vi "ResultsViewer.vi"(8 "Error in":errorcluster, 11 "TDMS path":path=path "") -> (0 "Error out":errorcluster)   [LabVIEW 2019]
panel:
  out "Loaded TDMS Filename":string
  out "O2 Saturation":dbl[](graph)
  out "Heart beat":dbl[](graph)
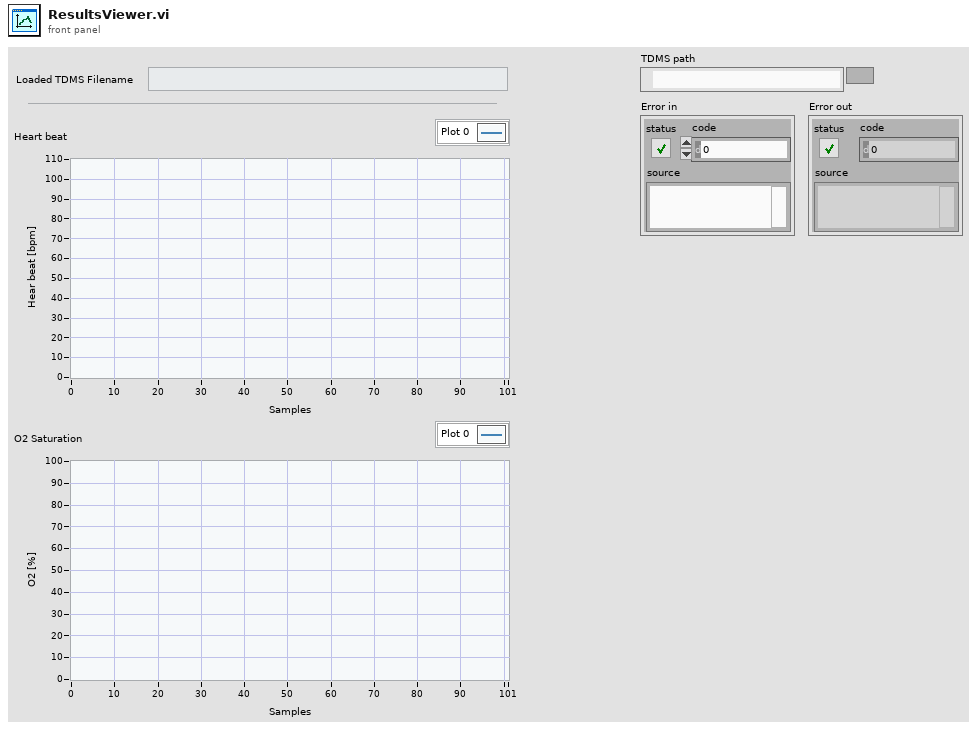
[diagram p1: front panel]
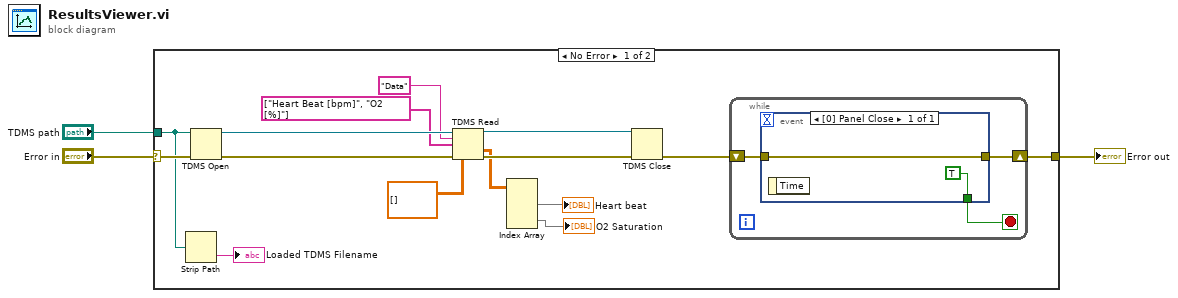
[diagram p0: block diagram]
diagram:
  n1 = case shown="No Error" "Error in" {
    selector: "Error in" -> [w6 w24]
    tunnel: [w17 w24] -> w3
    tunnel: "TDMS path" -> [w5 _]
    frame No Error {
      n2 = Strip Path(path=w5) -> (name=→"Loaded TDMS Filename":string)  [unwired: 1 out]
      n3 = TDMS Open(8:w6, 11:w5) -> (0:w15:errorcluster, 3:w16:refnum<k34>)  [unwired: 5 in]
      n4 = TDMS Read(0:w16, 5:"Data" ("group name in (Untitled)"), 7:string[] ["Heart Beat [bpm]", "O2 [%]"] ("channel name(s) in (Untitled)"), 11:w15, 12:dbl[][] []) -> (4:w14:refnum<k34>, 10:w9:dbl[][], 15:w13:errorcluster)  [unwired: 3 in, 3 out]
      n5 = Index Array(array=w9) -> (element #1=→"Heart beat":dbl[], element #2=→"O2 Saturation":dbl[])  [unwired: 4 in]
      n6 = TDMS Close(8:w13, 11:w14) -> (0:w18:errorcluster)  [unwired: 1 out]
      n7 = while {
        shift-right: [w19] -> w17
        shift-left: w18 -> [w21]
        stop <- w20 stop-if-true
        n8 = event shown="[0] Panel Close" {
          selector: _ -> [_]
          dyn-events: _ -> [_]
          timeout: _ -> [_]
          tunnel: w21 -> [w22]
          tunnel: [TRUE] -> w20
          tunnel: [w22] -> w19
          event Panel Close {
            n9 = event-data() -> ()  [unwired: 1 in, 1 out]
          }
        }
      }
    }
    frame Error {
    }
  }
  "Error out" <- w3
